vi "Execute Command.vi"(6 "Arguments":string[](array[string]), 8 "error in (no error)":errorcluster, 9 "File Paths":path[](array[path]), 10 "Command":string, 11 "Git Implementation in":refnum<class "Git Implementation.lvclass">) -> (0 "error out":errorcluster, 2 "CMD Return":T1, 3 "Git Implementation out":refnum<class "Git Implementation.lvclass">)   [LabVIEW 2017, in "Git-LabVIEW.lvlib" / "Git Implementation.lvclass"]
uses:
  Git Implementation.lvclass
  CMD Return.ctl
  Git Implementation.lvclass/Git Implementation.ctl
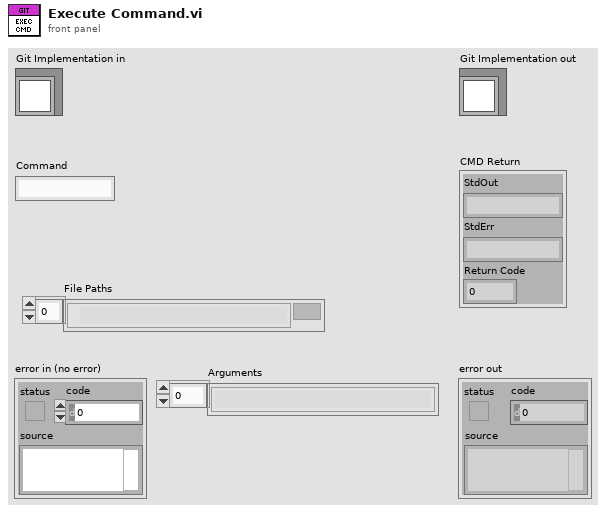
[diagram p1: front panel]
types:
  T1 = typedef "Git-LabVIEW.lvlib/Git Implementation.lvclass/CMD Return.ctl" = cluster{"StdOut":string, "StdErr":string, "Return Code":i32}
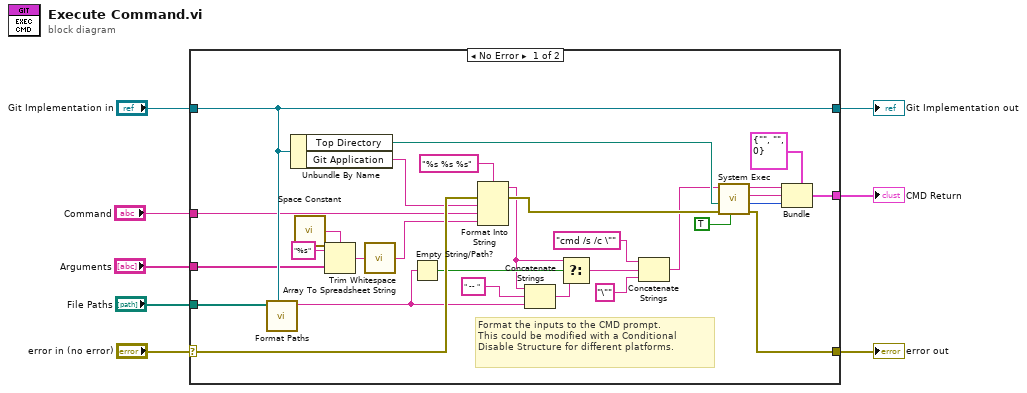
[diagram p0: block diagram]
diagram:
  n1 = case shown="No Error" "error in (no error)" {
    selector: "error in (no error)" -> [w36 w39]
    tunnel: [w29 w39] -> w7
    tunnel: [w37 w38] -> w5
    tunnel: "Git Implementation in" -> [w37 w38]
    tunnel: "Arguments" -> [w33 _]
    tunnel: "File Paths" -> [w31 _]
    tunnel: "Command" -> [w26 _]
    tunnel: [w12 _] -> w1
    frame No Error {
      # "Format the inputs to the CMD prompt.\nThis could be modified with a Conditional Disable Structure for different platforms."
      n2 = call-dynamic "Format Paths.vi"("Git Implementation in"=w37, "File Paths"=w31) -> ("Formatted Path String"=w9:string)  [unwired: 9 in]
      n3 = Unbundle By Name(w37) -> ("Top Directory"=w35:path, "Git Application"=w17:string)
      n4 = call <vilib>:"Space Constant.vi"() -> ("String"=w30:string)
      n5 = Array To Spreadsheet String(delimiter (Tab)=w30, array=w33, 3:"%s") -> (spreadsheet string=w32:string)
      n6 = call <vilib>:"Trim Whitespace.vi"("string"=w32) -> ("trimmed string"=w10:string)  [unwired: 1 in]
      n7 = Empty String/Path?(string/path=w9) -> (empty?=w24:bool)
      n8 = Format Into String(format string="%s %s %s", error in=w36, w17, w26, w10) -> (resulting string=w21:string, error out=w28:errorcluster)  [unwired: 1 in]
      n9 = Concatenate Strings(w21, " -- " ("string"), w9) -> (w22:string)
      n10 = Select(t=w21, s=w24, f=w22) -> (s? t:f=w19:string)
      n11 = Concatenate Strings("cmd /s /c \"" ("command line"), w19, "\"" ("string")) -> (w18:string)
      n12 = call <vilib>:"System Exec.vi"("run minimized? (F)"=TRUE, "error in (no error)"=w28, "working directory"=w35, "command line"=w18) -> ("error out"=w29:errorcluster, "return code"=w13:i32, "standard error"=w14:string, "standard output"=w15:string)  [unwired: 4 in]
      n13 = Bundle(cluster=T1 {"StdOut"="", "StdErr"="", "Return Code"=0} ("CMD Return"), "StdOut"=w15, "StdErr"=w14, "Return Code"=w13) -> (w12:T1)
    }
    frame Error {
    }
  }
  "error out" <- w7
  "Git Implementation out" <- w5
  "CMD Return" <- w1
